vi "Send Data Handshake.vi"(0 "READY":bool, 12 "first iteration in this state?":bool) -> (4 "VALID":bool, 6 "done?":bool)   [LabVIEW 2015, in "niInstr AXI4-Lite - FXP32 Address - FXP32 Data v1 FPGA.lvclass"]
doc: "Controls the logic of when data is valid, based on the <b>READY</b> signal.\n\n<B>Input Parameters</B>\n\n<B>READY</B> indicates that the signal is ready to be written or read.\n\n<B>first iteration in this state?</B> is true on the first clock cycle that the bus interface was in the current state.\n\n<B>Output Parameters</B>\n\n<B>VALID</B> is true while data is in the process of being transferred. When the transfer completes, it deasserts.\n\n<B>done?</B> asserts when the transfer completes. It will stay asserted until 'first iteration in this state?' is asserted and READY is not asserted on that same clock cycle."
uses:
  <instrlib>/_niInstr/CLIP Adapters/v1/FPGA/AXI4-Lite/FXP32 Address - FXP32 Data/niInstr AXI4-Lite - FXP32 Address - FXP32 Data v1 FPGA.lvclass
  <instrlib>/_niInstr/Basic Elements/v1/FPGA/niInstr Basic Elements v1 FPGA.lvlib
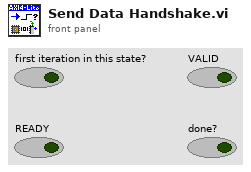
[diagram p1: front panel]
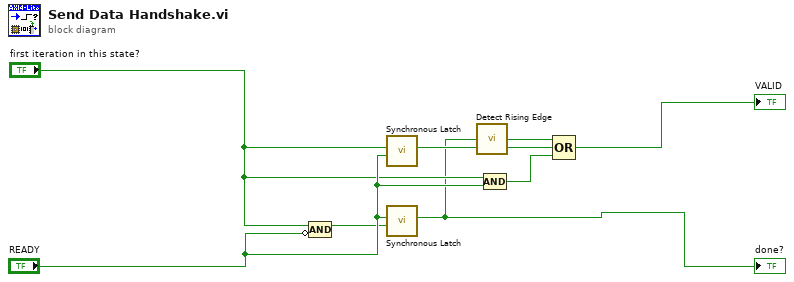
[diagram p0: block diagram]
diagram:
  n1 = Compound Arithmetic op=AND("first iteration in this state?", invert "READY") -> (w4:bool)
  n2 = call <instrlib>:"Synchronous Latch.vi"("clear"="READY", "set"="first iteration in this state?") -> ("out"=w5:bool)  [unwired: 9 in]
  n3 = call <instrlib>:"Synchronous Latch.vi"("clear"=w4, "set"="READY") -> ("out"=w1:bool)  [unwired: 9 in]
  "done?" <- w1
  n4 = call <instrlib>:"Detect Rising Edge.vi"("signal"=w1) -> ("edge detected"=w2:bool)  [unwired: 14 in]
  n5 = Compound Arithmetic op=AND("first iteration in this state?", "READY") -> (w3:bool)
  n6 = Compound Arithmetic op=OR(w2, w5, w3) -> (→"VALID":bool)
